vi "GetXYSetPoints.vi"(8 "error in (no error)":errorcluster, 11 "Asylum_Driver in":refnum<class "Asylum_Driver.lvclass">) -> (0 "error out":errorcluster, 1 "Y PIS Controls":T1, 2 "X PIS Controls":T1, 3 "Asylum_Driver out":refnum<class "Asylum_Driver.lvclass">)   [LabVIEW 2019, in "Asylum_Driver.lvclass"]
uses:
  Asylum_Driver.lvclass
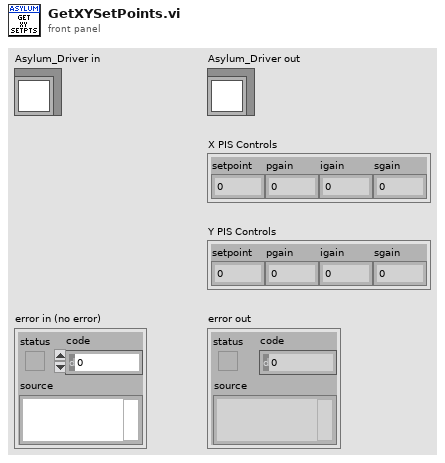
[diagram p1: front panel]
types:
  T1 = cluster{"setpoint":dbl, "pgain":dbl, "igain":dbl, "sgain":dbl}
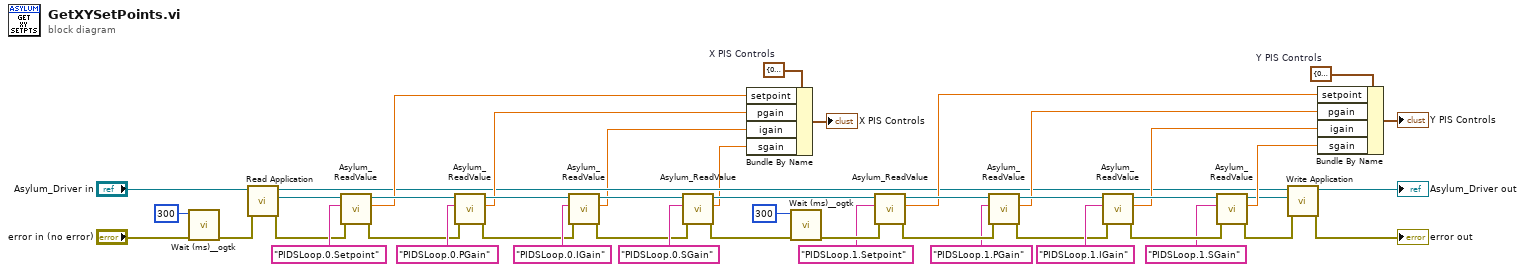
[diagram p0: block diagram]
diagram:
  w36 = T1 {"setpoint"=0.0, "pgain"=0.0, "igain"=0.0, "sgain"=0.0}  # Y PIS Controls
  w44 = T1 {"setpoint"=0.0, "pgain"=0.0, "igain"=0.0, "sgain"=0.0}  # X PIS Controls
  n1 = call <userlib>:"Wait (ms)__ogtk.vi"("error in (no error)"="error in (no error)", "milliseconds to wait"=u32 300) -> ("error out"=w8:errorcluster)  [unwired: 8 in, 1 out]
  n2 = call-dynamic "Read Application.vi"("error in (no error)"=w8, "Asylum_Driver in"="Asylum_Driver in") -> ("error out"=w7:errorcluster, "Application"=w15:refnum<k7>)  [unwired: 7 in, 1 out]
  n3 = call <userlib>:"Asylum_ReadValue.vi"("error in (no error)"=w7, "Value"="PIDSLoop.0.Setpoint", "Application"=w15) -> ("error out"=w3:errorcluster, "Value"=w37:dbl, "Application"=w43:refnum<k7>)  [unwired: 6 in]
  n4 = call <userlib>:"Asylum_ReadValue.vi"("error in (no error)"=w3, "Value"="PIDSLoop.0.PGain", "Application"=w43) -> ("error out"=w4:errorcluster, "Value"=w38:dbl, "Application"=w42:refnum<k7>)  [unwired: 6 in]
  n5 = call <userlib>:"Asylum_ReadValue.vi"("error in (no error)"=w4, "Value"="PIDSLoop.0.IGain", "Application"=w42) -> ("error out"=w5:errorcluster, "Value"=w1:dbl, "Application"=w41:refnum<k7>)  [unwired: 6 in]
  n6 = call <userlib>:"Asylum_ReadValue.vi"("error in (no error)"=w5, "Value"="PIDSLoop.0.SGain", "Application"=w41) -> ("error out"=w6:errorcluster, "Value"=w2:dbl, "Application"=w28:refnum<k7>)  [unwired: 6 in]
  n7 = Bundle By Name(cluster=w44, "setpoint"=w37, "pgain"=w38, "igain"=w1, "sgain"=w2) -> (→"X PIS Controls":T1)
  n8 = call <userlib>:"Wait (ms)__ogtk.vi"("error in (no error)"=w6, "milliseconds to wait"=u32 300) -> ("error out"=w23:errorcluster)  [unwired: 8 in, 1 out]
  n9 = call <userlib>:"Asylum_ReadValue.vi"("error in (no error)"=w23, "Value"="PIDSLoop.1.Setpoint", "Application"=w28) -> ("error out"=w32:errorcluster, "Value"=w27:dbl, "Application"=w29:refnum<k7>)  [unwired: 6 in]
  n10 = call <userlib>:"Asylum_ReadValue.vi"("error in (no error)"=w32, "Value"="PIDSLoop.1.PGain", "Application"=w29) -> ("error out"=w33:errorcluster, "Value"=w22:dbl, "Application"=w30:refnum<k7>)  [unwired: 6 in]
  n11 = call <userlib>:"Asylum_ReadValue.vi"("error in (no error)"=w33, "Value"="PIDSLoop.1.IGain", "Application"=w30) -> ("error out"=w34:errorcluster, "Value"=w26:dbl, "Application"=w31:refnum<k7>)  [unwired: 6 in]
  n12 = call <userlib>:"Asylum_ReadValue.vi"("error in (no error)"=w34, "Value"="PIDSLoop.1.SGain", "Application"=w31) -> ("error out"=w11:errorcluster, "Value"=w25:dbl, "Application"=w12:refnum<k7>)  [unwired: 6 in]
  n13 = call-dynamic "Write Application.vi"("error in (no error)"=w11, "Application"=w12, "Asylum_Driver in"="Asylum_Driver in") -> ("error out"=→"error out":errorcluster, "Asylum_Driver out"=→"Asylum_Driver out":refnum<class "Asylum_Driver.lvclass">)  [unwired: 7 in]
  n14 = Bundle By Name(cluster=w36, "setpoint"=w27, "pgain"=w22, "igain"=w26, "sgain"=w25) -> (→"Y PIS Controls":T1)
